vi "check-if-in-array.vi"(10 "tool# or drive subsystem name":string, 11 "Tool array in":T1[](array[typedef])) -> (2 "Position if found":i32, 3 "Found?":bool)   [LabVIEW 2017, in "labview-standard-library.lvlib" / "automode-scripting.lvlib"]
uses:
  automode-scripting.lvlib
  type-defs/tool-call-tracker.ctl
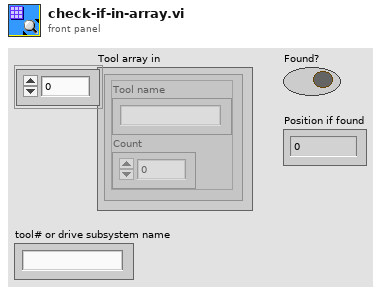
[diagram p1: front panel]
types:
  T1 = typedef "tool-call-tracker.ctl" = cluster{"Tool name":string, "Count":i32}
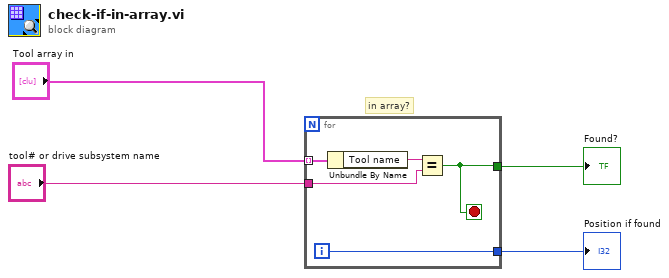
[diagram p0: block diagram]
diagram:
  # "in array?"
  n1 = for {
    tunnel: "Tool array in" -> [w9] mode=indexing
    tunnel: "tool# or drive subsystem name" -> [w7]
    tunnel: [w6] -> w1
    tunnel: [w5] -> w4
    i -> [w5]
    stop <- w6 stop-if-true
    n2 = Unbundle By Name(w9) -> ("Tool name"=w8:string)
    n3 = Equal?(x=w8, y=w7) -> (x = y?=w6:bool)
  }
  "Position if found" <- w4
  "Found?" <- w1
